vi "FolderMon catalog.vi"(4 "error in (no error)":errorcluster, 7 "Folder":path) -> (0 "error out":errorcluster, 1 "Any Changes?":bool, 2 "Changes":T3)   [LabVIEW 2011]
uses:
  FolderMon changes.ctl
panel:
  out "Array":T1(array[cluster])
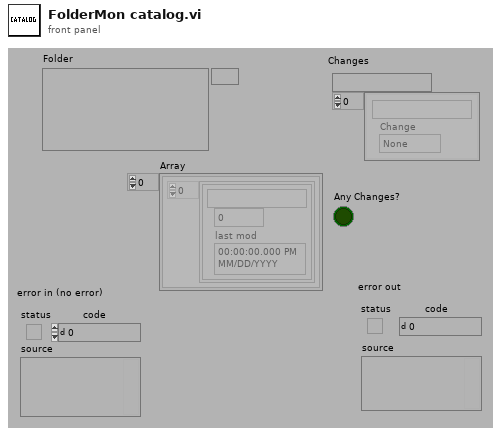
[diagram p1: front panel]
types:
  T1 = cluster{cluster{string, i32, "last mod":timestamp}[]}[]
  T2 = typedef "FolderMon changes.ctl" = enum16{"None", "First", "New", "Properties", "Deleted"}
  T3 = cluster{"Folder":path, "Changed Files":cluster{string, "Change":T2}[]}
  T4 = cluster{cluster{string, i32, "last mod":timestamp}[]}
  T5 = cluster{"path out":path, cluster{string, "Change":T2}[]}
  T6 = cluster{"path out":path, "Changed Files":cluster{"File":string, "Change":T2}[]}
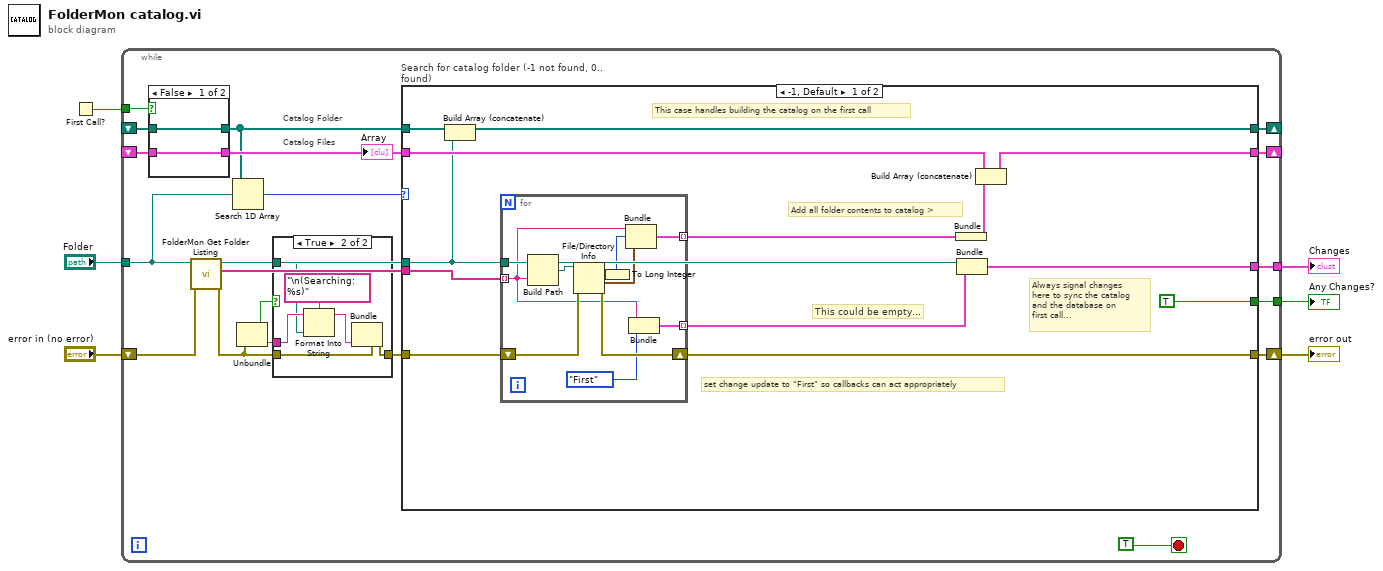
[diagram p0: block diagram]
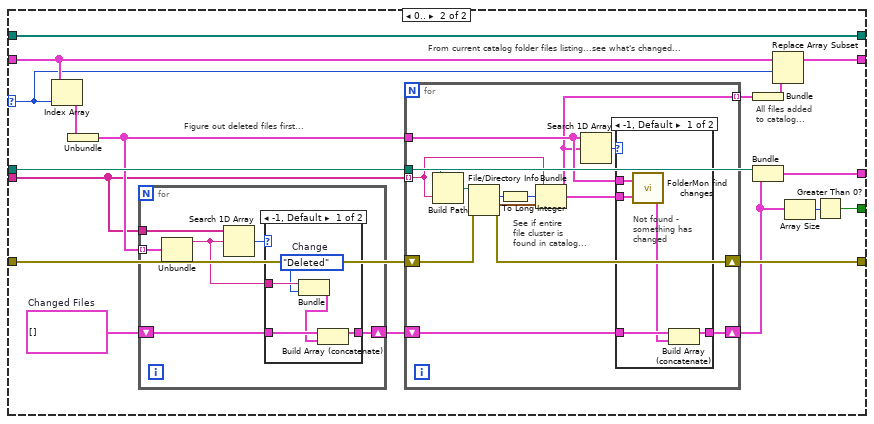
[diagram p4: hidden frame]
diagram:
  n1 = First Call?() -> (First Call?: T/F=w2:bool)
  n2 = while {
    shift-right: [w24] -> w5
    shift-left: "error in (no error)" -> [w13]
    shift-right: [w25] -> _
    shift-left: _ -> [w10]
    shift-right: [w23] -> _
    shift-left: _ -> [w9]
    tunnel: [w22] -> w4
    tunnel: [w20] -> w3
    tunnel: "Folder" -> [w15]
    tunnel: w2 -> [w11]
    stop <- TRUE stop-if-true
    # "Catalog Files"
    # "Catalog Folder"
    n3 = case shown="False" w11 {
      tunnel: w10 -> [w27 _]
      tunnel: w9 -> [w28 _]
      tunnel: [w28 _] -> w8
      tunnel: [w27 _] -> w7
      frame False {
      }
      frame True {
      }
    }
    "Array" <- w8
    n4 = call "FolderMon Get Folder Listing.vi"("error in (no error)"=w13, "Path"=w15) -> ("error out"=w12:errorcluster, "file names"=w14:string[], "path out"=w16:path)  [unwired: 7 out]
    n5 = Search 1D Array(1D array=w7, element=w15) -> (index of element=w26:i32)  [unwired: 1 out]
    n6 = Unbundle(w12) -> ("status"=w17:bool, "source"=w18:string)  [unwired: 1 out]
    n7 = case shown="True" w17 {
      tunnel: w12 -> [w29 w35]
      tunnel: [w29 w34] -> w19
      tunnel: w16 -> [_ w31]
      tunnel: w18 -> [_ w33]
      frame False {
      }
      frame True {
        n8 = Format Into String(format string="\n(Searching: %s)" ("string"), initial string=w33, w31) -> (resulting string=w30:string)  [unwired: 1 in, 1 out]
        n9 = Bundle(cluster=w35, "source"=w30) -> (w34:errorcluster)  [unwired: 2 out]
      }
    }
    n10 = case "Search for catalog folder (-1 not found, 0.. found)" shown="-1, Default" w26 {
      selector: w26 -> [_ w70]
      tunnel: w19 -> [w46 w69]
      tunnel: w7 -> [w48 w77]
      tunnel: w14 -> [w45 w64]
      tunnel: w16 -> [w39 w67]
      tunnel: [w47 w77] -> w25
      tunnel: [w44 w68] -> w24
      tunnel: w8 -> [w43 w74]
      tunnel: [w40 w73] -> w23
      tunnel: [w38 w75] -> w22
      tunnel: [TRUE w60] -> w20
      frame -1, Default {
        # "This could be empty..."
        # "Always signal changes \nhere to sync the catalog\nand the database on\nfirst call..."
        # "Add all folder contents to catalog >"
        # "set change update to \"First\" so callbacks can act appropriately"
        # "This case handles building the catalog on the first call"
        n11 = Build Array (concatenate)(w48, w39) -> (w47:path[])
        n12 = for {
          tunnel: w39 -> [w59]
          shift-right: [w56] -> w44
          shift-left: w46 -> [w57]
          tunnel: w45 -> [w52] mode=indexing
          tunnel: [w53] -> w42 mode=indexing
          tunnel: [w50] -> w37 mode=indexing
          n13 = Build Path(base path=w59, name or relative path=w52) -> (appended path=w58:path)
          n14 = File/Directory Info(path=w58, error in=w57) -> (size=w49:i64, last mod=w54:timestamp, error out=w56:errorcluster)  [unwired: 4 out]
          n15 = To Long Integer(number=w49) -> (32bit integer=w55:i32)
          n16 = Bundle(w52, w55, "last mod"=w54) -> (w53:cluster{string, i32, "last mod":timestamp})  [unwired: 1 out]
          n17 = Bundle(w52, "Change"=FolderMon_changes."First") -> (w50:cluster{string, "Change":T2})  [unwired: 1 out]
        }
        n18 = Bundle(w42) -> (w41:T4)  [unwired: 1 in]
        n19 = Bundle("path out"=w39, w37) -> (w38:T5)  [unwired: 1 out]
        n20 = Build Array (concatenate)(w43, w41) -> (w40:T1)
      }
      frame 0.. {
        w65 = cluster{"File":string, "Change":T2}[] []  # Changed Files
        # "All files added\nto catalog..."
        # "From current catalog folder files listing...see what's changed..."
        # "Figure out deleted files first..."
        n21 = Index Array(array=w74, index=w70) -> (element=w76:T4)
        n22 = Unbundle(w76) -> (w66:cluster{string, i32, "last mod":timestamp}[])
        n23 = for {
          shift-right: [w81] -> w63
          shift-left: w65 -> [w83]
          tunnel: w66 -> [w80] mode=indexing
          tunnel: w64 -> [w79]
          n24 = Unbundle(w80) -> (w78:string)  [unwired: 2 out]
          n25 = Search 1D Array(1D array=w79, element=w78) -> (index of element=w82:i32)  [unwired: 1 out]
          n26 = case shown="-1, Default" w82 {
            tunnel: w83 -> [w87 w89]
            tunnel: [w88 w89] -> w81
            tunnel: w78 -> [w86 _]
            frame -1, Default {
              w85 = FolderMon_changes."Deleted"  # Change
              n27 = Bundle(w86, "Change"=w85) -> (w84:cluster{string, "Change":T2})  [unwired: 1 out]
              n28 = Build Array (concatenate)(w87, w84) -> (w88:cluster{"File":string, "Change":T2}[])
            }
            frame 0.. {
            }
          }
        }
        n29 = for {
          tunnel: w66 -> [w99]
          shift-right: [w100] -> w61
          shift-left: w63 -> [w102]
          tunnel: [w91] -> w72 mode=indexing
          shift-right: [w94] -> w68
          shift-left: w69 -> [w95]
          tunnel: w67 -> [w93]
          tunnel: w64 -> [w92] mode=indexing
          # "See if entire\nfile cluster is\nfound in catalog..."
          n30 = Build Path(base path=w93, name or relative path=w92) -> (appended path=w96:path)
          n31 = File/Directory Info(path=w96, error in=w95) -> (size=w90:i64, last mod=w98:timestamp, error out=w94:errorcluster)  [unwired: 4 out]
          n32 = To Long Integer(number=w90) -> (32bit integer=w97:i32)
          n33 = Bundle(w92, w97, "last mod"=w98) -> (w91:cluster{string, i32, "last mod":timestamp})  [unwired: 1 out]
          n34 = Search 1D Array(1D array=w99, element=w91) -> (index of element=w101:i32)  [unwired: 1 out]
          n35 = case shown="-1, Default" w101 {
            tunnel: w102 -> [w106 w108]
            tunnel: [w107 w108] -> w100
            tunnel: w91 -> [w103 _]
            tunnel: w99 -> [w104 _]
            frame -1, Default {
              # "Not found -\nsomething has\nchanged"
              n36 = call "FolderMon find changes.vi"("Current File"=w103, "All Historic Files"=w104) -> ("Changed File"=w105:cluster{"File":string, "Change":T2})
              n37 = Build Array (concatenate)(w106, w105) -> (w107:cluster{"File":string, "Change":T2}[])
            }
            frame 0.. {
              # "It's found -\nno changes\nwere made"
            }
          }
        }
        n38 = Bundle(w72) -> (w71:T4)  [unwired: 1 in]
        n39 = Bundle("path out"=w67, "Changed Files"=w61) -> (w75:T6)  [unwired: 1 out]
        n40 = Replace Array Subset(array=w74, new element=w71, index=w70) -> (w73:T1)
        n41 = Array Size(array=w61) -> (size(s)=w62:i32)
        n42 = Greater Than 0?(x=w62) -> (x > 0?=w60:bool)
      }
    }
  }
  "error out" <- w5
  "Changes" <- w4
  "Any Changes?" <- w3
